vi "double-is pythagorean.vi"(8 "error in (no error)":errorcluster, 11 "(a, b) in":T2) -> (0 "error out":errorcluster, 1 "Pythagorean triplet":T1, 2 "T = this double is Pythagorean (a^2+b^2=c^2)":bool, 3 "(a, b) out (duplicate)":T2)   [LabVIEW 2021, in "Project Euler.lvlib"]
uses:
  Project Euler.lvlib
  cluster-double.ctl
  cluster-triplet.ctl
panel:
  # "Development\ncontrols/indicators useful for development and testing, but which are not outputs of the VI"
  # "Input\nInputs to the VI"
  # "Output\nOutputs of the VI"
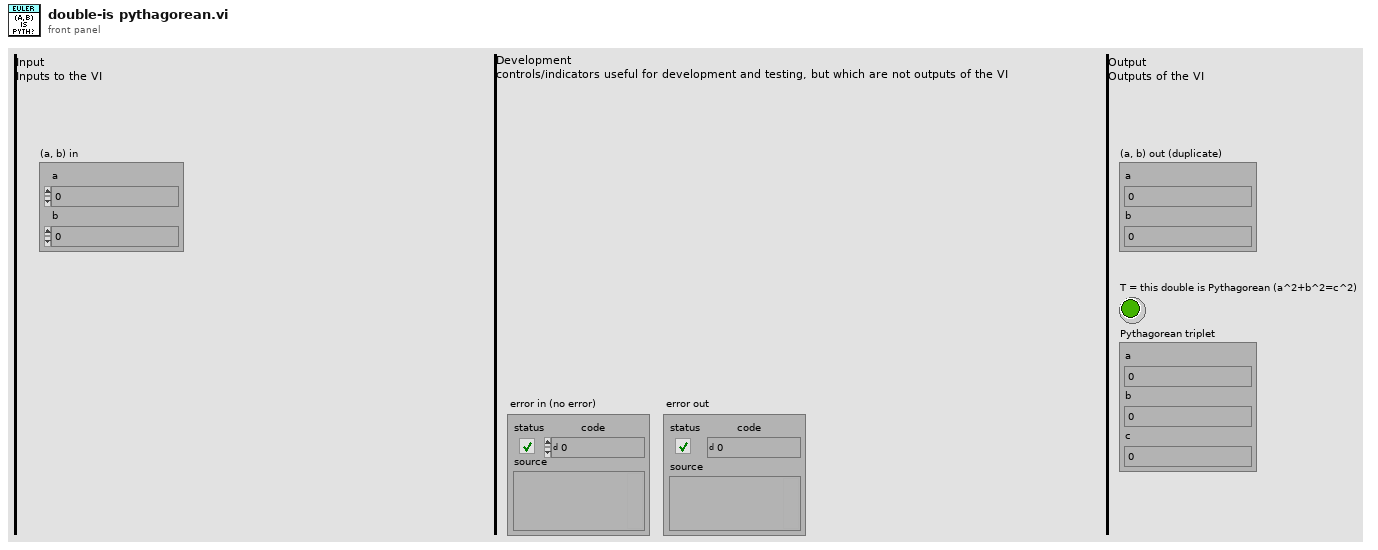
[diagram p1: front panel]
types:
  T1 = typedef "Project Euler.lvlib/cluster-triplet.ctl" = cluster{"a":i32, "b":i32, "c":i32}
  T2 = typedef "Project Euler.lvlib/cluster-double.ctl" = cluster{"a":i32, "b":i32}
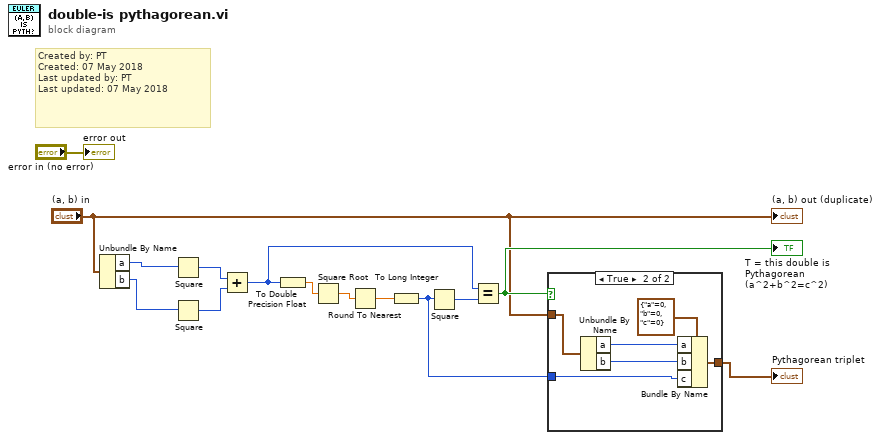
[diagram p0: block diagram]
diagram:
  # "Created by: PT\nCreated: 07 May 2018\nLast updated by: PT\nLast updated: 07 May 2018"
  n1 = Unbundle By Name("(a, b) in") -> ("a"=w13:i32, "b"=w12:i32)
  n2 = Square(x=w13) -> (x^2=w11:i32)
  n3 = Square(x=w12) -> (x^2=w10:i32)
  n4 = Add(x=w11, y=w10) -> (x+y=w5:i32)
  n5 = To Double Precision Float(number=w5) -> (double precision float=w9:dbl)
  n6 = Square Root(x=w9) -> (sqrt(x)=w8:dbl)
  n7 = Round To Nearest(number=w8) -> (nearest integer value=w7:dbl)
  n8 = To Long Integer(number=w7) -> (32bit integer=w1:i32)
  n9 = Square(x=w1) -> (x^2=w6:i32)
  n10 = Equal?(x=w5, y=w6) -> (x = y?=w4:bool)
  "T = this double is Pythagorean (a^2+b^2=c^2)" <- w4
  n11 = case shown="True" w4 {
    tunnel: "(a, b) in" -> [_ w19]
    tunnel: [_ w16] -> w2
    tunnel: w1 -> [_ w15]
    frame False {
    }
    frame True {
      n12 = Unbundle By Name(w19) -> ("a"=w18:i32, "b"=w17:i32)
      n13 = Bundle By Name(cluster=T1 {"a"=0, "b"=0, "c"=0} ("Pythagorean triplet"), "a"=w18, "b"=w17, "c"=w15) -> (w16:T1)
    }
  }
  "Pythagorean triplet" <- w2
  "error out" <- "error in (no error)"
  "(a, b) out (duplicate)" <- "(a, b) in"
